vi "R1C_TRX_Att.vi"(4 "Offset_Idle_OP":u32[](array[numeric]), 5 "RF":T2 items=["RF_0", "RF_1", "RF_2", "RF_3"], 6 "Offset_Reg_Data":u32[](array[numeric]), 7 "RFU":T1, 8 "Error_In":errorcluster, 9 "Auto_Sel_Rsrc?":bool=TRUE, 10 "Att":T3 items=["0.0", "0.5", "1.0", "1.5", "2.0", "2.5", "3.0", "3.5", "4.0", "4.5", "5.0", "5.5", "6.0", "6.5", "7.0", "7.5", "8.0", "8.5", "9.0", "9.5", "10.0", "10.5", "11.0", "11.5", "12.0", "12.5", "13.0", "13.5", "14.0", "14.5", "15.0", "15.5", "16.0", "16.5", "17.0", "17.5", "18.0", "18.5", "19.0", "19.5", "20.0", "20.5", "21.0", "21.5", "22.0", "22.5", "23.0", "23.5", "24.0", "24.5", "25.0", "25.5", "26.0", "26.5", "27.0", "27.5", "28.0", "28.5", "29.0", "29.5", "30.0", "30.5", "31.0", "31.5"], 11 "VISA_Rsrc_In":refnum<visa-resource-name>) -> (0 "Error_Out":errorcluster, 3 "VISA_Rsrc_Out":refnum<visa-resource-name>)   [LabVIEW 2018]
uses:
  Types/Att(0-0.5-31.5).ctl
  Types/RF.ctl
  Types/RFU.ctl
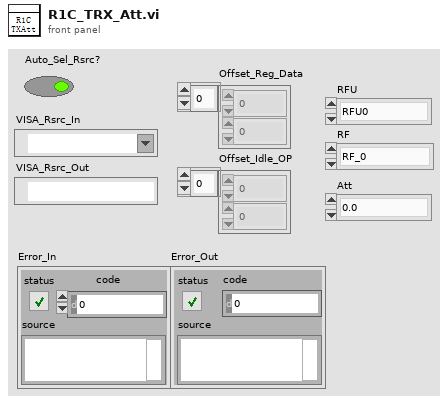
[diagram p1: front panel]
types:
  T1 = typedef "RFU.ctl" = enum8{"RFU0", "RFU1", "RFU2", "RFU3", "RFU4"}
  T2 = typedef "RF.ctl" = u16
  T3 = typedef "Att(0-0.5-31.5).ctl" = dbl
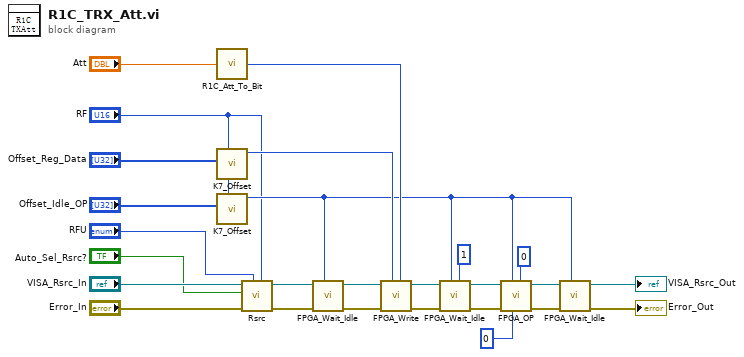
[diagram p0: block diagram]
diagram:
  n1 = call "R1C_Att_To_Bit.vi"("Att"="Att") -> ("Bit"=w25:u32)
  n2 = call "K7_Offset.vi"("RF"="RF", "Offset"="Offset_Reg_Data") -> ("Offset"=w18:u32)  [unwired: 9 in]
  n3 = call "K7_Offset.vi"("RF"="RF", "Offset"="Offset_Idle_OP") -> ("Offset"=w15:u32)  [unwired: 9 in]
  n4 = call "Rsrc.vi"("RF"="RF", "RFU"="RFU", "Error_In"="Error_In", "Auto_Sel_Rsrc?"="Auto_Sel_Rsrc?", "VISA_Rsrc_In"="VISA_Rsrc_In") -> ("Error_Out"=w1:errorcluster, "VISA_Rsrc_Out"=w2:refnum<visa-resource-name>)  [unwired: 5 in]
  n5 = call "FPGA_Wait_Idle.vi"("Offset"=w15, "Error_In"=w1, "VISA_Rsrc_In"=w2) -> ("Error_Out"=w23:errorcluster, "VISA_Rsrc_Out"=w24:refnum<visa-resource-name>)  [unwired: 7 in]
  n6 = call "FPGA_Write.vi"("Value"=w25, "Offset"=w18, "Error_In"=w23, "VISA_Rsrc_In"=w24) -> ("Error_Out"=w21:errorcluster, "VISA_Rsrc_Out"=w22:refnum<visa-resource-name>)  [unwired: 6 in]
  n7 = call "FPGA_Wait_Idle.vi"("Bit_Offset"=u32 1, "Offset"=w15, "Error_In"=w21, "VISA_Rsrc_In"=w22) -> ("Error_Out"=w19:errorcluster, "VISA_Rsrc_Out"=w20:refnum<visa-resource-name>)  [unwired: 6 in]
  n8 = call "FPGA_OP.vi"("Origin_Value"=u32 0, "OP_Offset"=u32 0, "Offset"=w15, "Error_In"=w19, "VISA_Rsrc_In"=w20) -> ("Error_Out"=w16:errorcluster, "VISA_Rsrc_Out"=w17:refnum<visa-resource-name>)  [unwired: 5 in]
  n9 = call "FPGA_Wait_Idle.vi"("Offset"=w15, "Error_In"=w16, "VISA_Rsrc_In"=w17) -> ("Error_Out"=→"Error_Out":errorcluster, "VISA_Rsrc_Out"=→"VISA_Rsrc_Out":refnum<visa-resource-name>)  [unwired: 7 in]
